vi "setData.vi"(8 "error in (no error)":errorcluster, 9 "Data":u8[](array[numeric]), 10 "Index":i32, 11 "FixedFrameBuilder in":refnum<class "FixedFrameBuilder.lvclass">) -> (0 "error out":errorcluster, 3 "FixedFrameBuilder out":refnum<class "FixedFrameBuilder.lvclass">)   [LabVIEW 2016, in "RTModbus.lvlib" / "FixedFrameBuilder.lvclass"]
uses:
  FixedFrameBuilder.lvclass
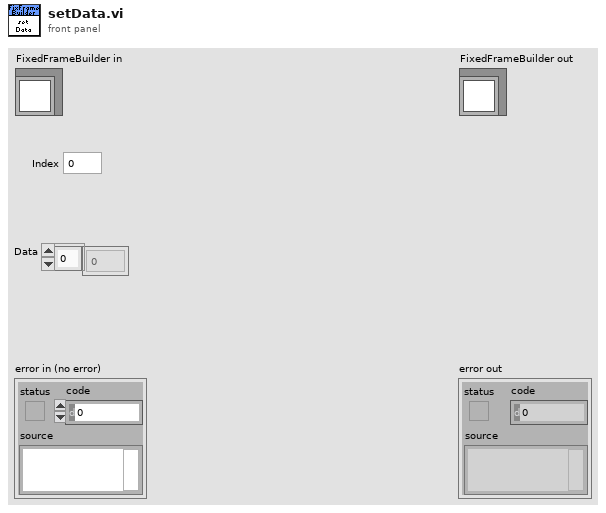
[diagram p1: front panel]
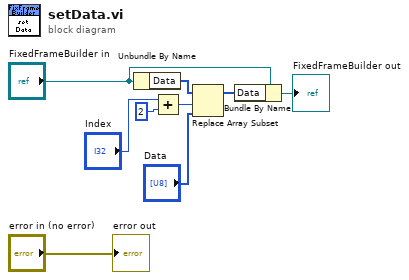
[diagram p0: block diagram]
diagram:
  n1 = Unbundle By Name("FixedFrameBuilder in") -> ("Data"=w9:u8[])
  n2 = Add(x="Index", y=2) -> (x+y=w1:i32)
  n3 = Replace Array Subset(array=w9, new element="Data", index=w1) -> (w6:u8[])
  n4 = Bundle By Name(cluster="FixedFrameBuilder in", "Data"=w6) -> (→"FixedFrameBuilder out":refnum<class "FixedFrameBuilder.lvclass">)
  "error out" <- "error in (no error)"
